vi "MGI Close Window.vi"(8 "error in (no error)":errorcluster, 11 "Open Initially?":bool) -> (0 "error out":errorcluster)   [LabVIEW 2016]
doc: "Closes the caller VI and sets its behavior to default (so it will not be modal anymore and thus you will not have problems getting stuck with it open). If you wire the Open Initially? input, then it will not close the VI if it was open initially (this is useful so that it doesn't close if you run it while working on it in the IDE).\n\nAuthor: Hope Harrison\nsupport@mooregoodideas.com\nwww.mooregoodideas.com\n\nCopyright (c) 2016, Moore Good Ideas, Inc.\n\nAll rights reserved.\n\nRedistribution and use in source and binary forms, with or without modification, are permitted provided that the following conditions are met:\n\n * Redistributions of source code must retain the above copyright notice, this list of conditions and the following disclaimer.\n * Redistributions in binary form must reproduce the above copyright notice, this list of conditions and the following disclaimer in the documentation and/or other materials provided with the distribution.\n * Neither the name of Moore Good Ideas, Inc. nor the names of its contributors may be used to endorse or promote products derived from this software without specific prior written permission.\n\nTHIS SOFTWARE IS PROVIDED BY THE COPYRIGHT HOLDERS AND CONTRIBUTORS \"AS IS\" AND ANY EXPRESS OR IMPLIED WARRANTIES, INCLUDING, BUT NOT LIMITED TO, THE IMPLIED WARRANTIES OF MERCHANTABILITY AND FITNESS FOR A PARTICULAR PURPOSE ARE DISCLAIMED. IN NO EVENT SHALL THE COPYRIGHT OWNER OR CONTRIBUTORS BE LIABLE FOR ANY DIRECT, INDIRECT, INCIDENTAL, SPECIAL, EXEMPLARY, OR CONSEQUENTIAL DAMAGES (INCLUDING, BUT NOT LIMITED TO, PROCUREMENT OF SUBSTITUTE GOODS OR SERVICES; LOSS OF USE, DATA, OR PROFITS; OR BUSINESS INTERRUPTION) HOWEVER CAUSED AND ON ANY THEORY OF LIABILITY, WHETHER IN CONTRACT, STRICT LIABILITY, OR TORT (INCLUDING NEGLIGENCE OR OTHERWISE) ARISING IN ANY WAY OUT OF THE USE OF THIS SOFTWARE, EVEN IF ADVISED OF THE POSSIBILITY OF SUCH DAMAGE."
uses:
  <userlib>/_MGI/Application Control/MGI VI Reference/MGI Caller's VI Reference.vi
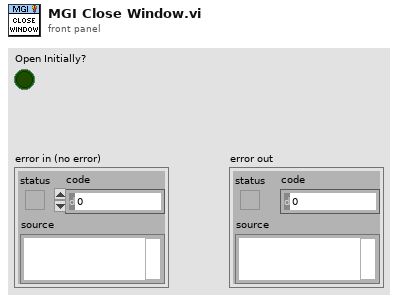
[diagram p1: front panel]
types:
  T1 = enum32{"Invalid", "Default", "Floating", "Floating/Auto-Hide", "Modal"}
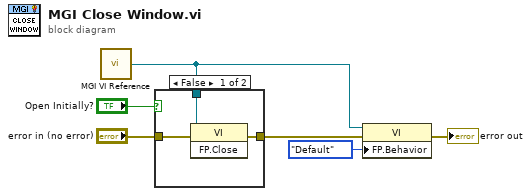
[diagram p0: block diagram]
diagram:
  n1 = call-poly <userlib>:"MGI VI Reference.vi"() -> ("Caller's VI Reference"=w1:refnum<vi>)  [unwired: 1 in]
  n2 = case shown="False" "Open Initially?" {
    tunnel: [w9 w10] -> w4
    tunnel: "error in (no error)" -> [w8 w10]
    tunnel: w1 -> [w7 _]
    frame False {
      n3 = invoke class="VI" method="FP.Close"(reference=w7, error in=w8) -> (error out=w9:errorcluster)  [unwired: 1 in, 2 out]
    }
    frame True {
    }
  }
  n4 = property class="VI"(reference=w1, error in=w4, "FP.Behavior"=T1."Default" ("Front Panel Window:Behavior")) -> (error out=→"error out":errorcluster)  [unwired: 1 out]
